vi "read timing source name.vi"(8 "error in":errorcluster, 11 "module in":refnum<class "Scan Engine runtime.lvclass">) -> (0 "error out":errorcluster, 2 "timing source":refnum<class "TBM timing source.lvclass">, 3 "module out":refnum<class "Scan Engine runtime.lvclass">)   [LabVIEW 2015, in "Scan Engine runtime.lvclass"]
uses:
  Scan Engine runtime.lvclass
  <vilib>/NI/Module Timing Source/timing source/TBM timing source.lvclass
  <vilib>/NI/Module Timing Source/scan engine timing source/scan engine timing source.lvclass
  Scan Engine runtime.lvclass/Scan Engine runtime.ctl
  <vilib>/NI/Module Timing Source/scan engine timing source/scan engine timing source.lvclass/scan engine timing source.ctl
  <vilib>/NI/Module Timing Source/scan engine timing source/Write scan period (uSec).vi
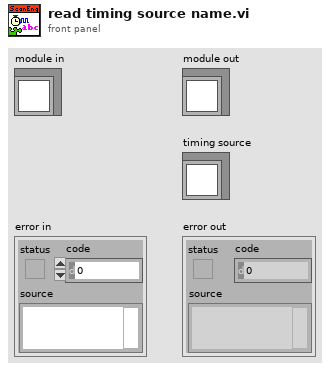
[diagram p1: front panel]
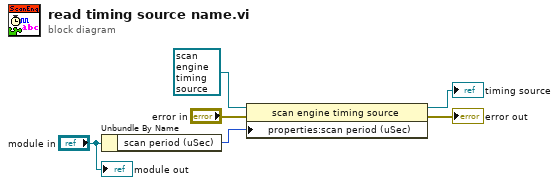
[diagram p0: block diagram]
diagram:
  n1 = Unbundle By Name("module in") -> ("scan period (uSec)"=w1:u32)
  n2 = property class="scan engine timing source"(reference=refnum<class "scan engine timing source.lvclass"> refnum ("scan engine timing source.lvclass"), error in="error in", "properties:scan period (uSec)"=w1) -> (reference out=→"timing source":refnum<class "scan engine timing source.lvclass">, error out=→"error out":errorcluster)
  "module out" <- "module in"
